vi "Test_Error_DeBounc.vi"() -> ()   [LabVIEW 2018]
panel:
  in  "s":bool
  out "Numeric":i32
  out "error out":errorcluster
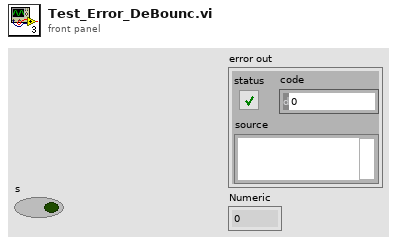
[diagram p1: front panel]
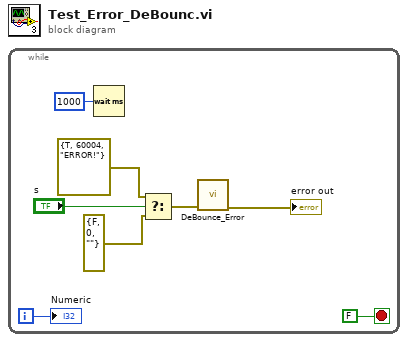
[diagram p0: block diagram]
diagram:
  n1 = while {
    i -> [w2]
    stop <- FALSE stop-if-true
    n2 = Wait (ms)(milliseconds to wait=u32 1000) -> ()  [unwired: 1 out]
    n3 = Select(t=errorcluster {"status"=TRUE, "code"=60004, "source"="ERROR!"} ("error constant"), s="s", f=errorcluster {"status"=FALSE, "code"=0, "source"=""} ("error constant")) -> (s? t:f=w4:errorcluster)
    n4 = call "DeBounce_Error.vi"("error in (no error)"=w4) -> ("error out"=→"error out":errorcluster)  [unwired: 10 in]
    "Numeric" <- w2
  }
